vi "OpenTcp.vi"(8 "error in (no error)":errorcluster, 11 "properties":T1[](array[typedef])) -> (0 "error out":errorcluster, 1 "read timeout (ms)":i32, 2 "read interval (sec)":dbl, 3 "serial master instance":refnum<class "Modbus Master.lvclass">)   [LabVIEW 2017, in "ModbusMaster.lvlib"]
uses:
  <vilib>/addons/InsightCM/Devices/Shared/Common/ModbusMaster/ModbusMaster.lvlib
  <vilib>/Modbus/master/Modbus Master.lvclass
  C:/Program Files (x86)/National Instruments/LabVIEW 2017/vi.lib/Modbus/subvis/Modbus API/Modbus API.lvclass
  <vilib>/addons/InsightCM/MessageBus/Base/controls/KeyValuePair.ctl
  <vilib>/Modbus/subvis/Modbus API/Modbus API.lvclass/Modbus API.ctl
  <vilib>/Modbus/subvis/Transmission Data Unit (ADU)/Transmission Data Unit/Transmission Data Unit.lvclass/Transmission Data Unit.ctl
  <vilib>/Modbus/master/Data Access/Unit ID/Set Unit ID Property.vi
  <vilib>/Modbus/subvis/Transmission Data Unit (ADU)/Transmission Data Unit/Data Access/Unit ID/Write Unit ID.vi
  <vilib>/Modbus/subvis/Modbus API/Read Transmission Data Unit.vi
  <vilib>/Modbus/subvis/Modbus API/Write Transmission Data Unit.vi
  <vilib>/Modbus/master/Create Master Instance (TCP).vi
  <vilib>/Modbus/subvis/Transmission Data Unit (ADU)/Transmission Data Unit/Transmission Data Unit.lvclass
  <vilib>/addons/InsightCM/Utilities/PropertyHelpers/PropertyHelpers.lvlib
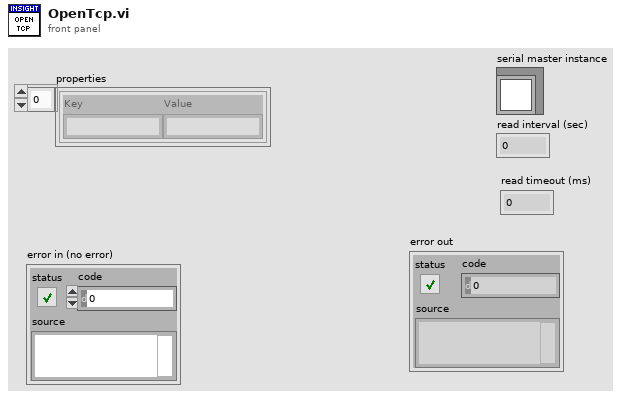
[diagram p1: front panel]
types:
  T1 = typedef "KeyValuePair.ctl" = cluster{"Key":string, "Value":string}
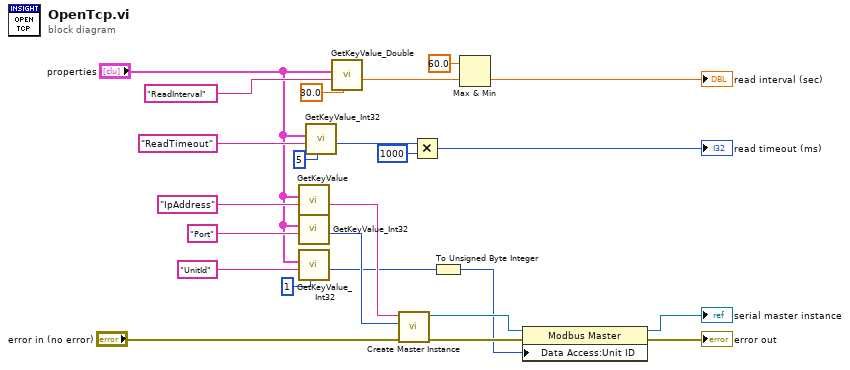
[diagram p0: block diagram]
diagram:
  n1 = call <vilib>:"GetKeyValue.vi"("key"="IpAddress", "key value pairs"="properties") -> ("value"=w23:string)  [unwired: 7 in, 2 out]
  n2 = call <vilib>:"GetKeyValue_Int32.vi"("key"="Port", "key value pairs"="properties") -> ("value"=w21:i32)  [unwired: 7 in, 2 out]
  n3 = call <vilib>:"GetKeyValue_Int32.vi"("default"=1, "key"="UnitId", "key value pairs"="properties") -> ("value"=w6:i32)  [unwired: 6 in, 2 out]
  n4 = call <vilib>:"GetKeyValue_Int32.vi"("default"=5, "key"="ReadTimeout", "key value pairs"="properties") -> ("value"=w15:i32)  [unwired: 6 in, 2 out]
  n5 = call <vilib>:"GetKeyValue_Double.vi"("default"=30.0, "key"="ReadInterval", "key value pairs"="properties") -> ("value"=w3:dbl)  [unwired: 6 in, 2 out]
  n6 = call-poly <vilib>:"Create Master Instance.vi"("error in (no error)"="error in (no error)", "port (502)"=w21, "address"=w23) -> ("error out"=w12:errorcluster, "TCP master instance"=w10:refnum<class "Modbus Master.lvclass">)  [unwired: 7 in]
  n7 = Multiply(x=w15, y=1000) -> (x*y=→"read timeout (ms)":i32)
  n8 = To Unsigned Byte Integer(number=w6) -> (unsigned 8bit integer=w5:u8)
  n9 = Max & Min(x=60.0, y=w3) -> (min(x,y)=→"read interval (sec)":dbl)  [unwired: 1 out]
  n10 = property class="Modbus Master"(reference=w10, error in=w12, "Data Access:Unit ID"=w5) -> (reference out=→"serial master instance":refnum<class "Modbus Master.lvclass">, error out=→"error out":errorcluster)
